vi "CreateLabview.vi"() -> ()   [LabVIEW 2015]
uses:
  Control_Function.ctl
panel:
  in  "Type_Frame":enum16{"SingelCaseFrame", "DoubleCaseFrame"}(ring)=enum."DoubleCaseFrame"
  in  "base path":path=path "D:/control"
  out "String":string
  out "output cluster":T1
  in  "Type_Enum":T2(ring)=enum."Constant"
  in  "Type_Buttom":enum16{"Cluster", "Control", "CheckBox"}(ring)=enum."Control"
  in  "初始化":bool
  in  "Path":path
  in  "初始化歸零?":bool
  in  "Value":string[][](array[string])
  in  "Name":string[](array[string])
  in  "Name_data":string
  in  "Data":string
  in  "檔案格式確認":bool
  in  "路徑修改":bool
  in  "讀出Data":bool
  in  "寫入Data":bool
  in  "結束":bool
  in  "製作框架":bool
  in  "製作按鈕":bool
  in  "儲存CSV":bool
  in  "讀取CSV":bool
  in  "儲存Control":bool
  in  "讀取Control":bool
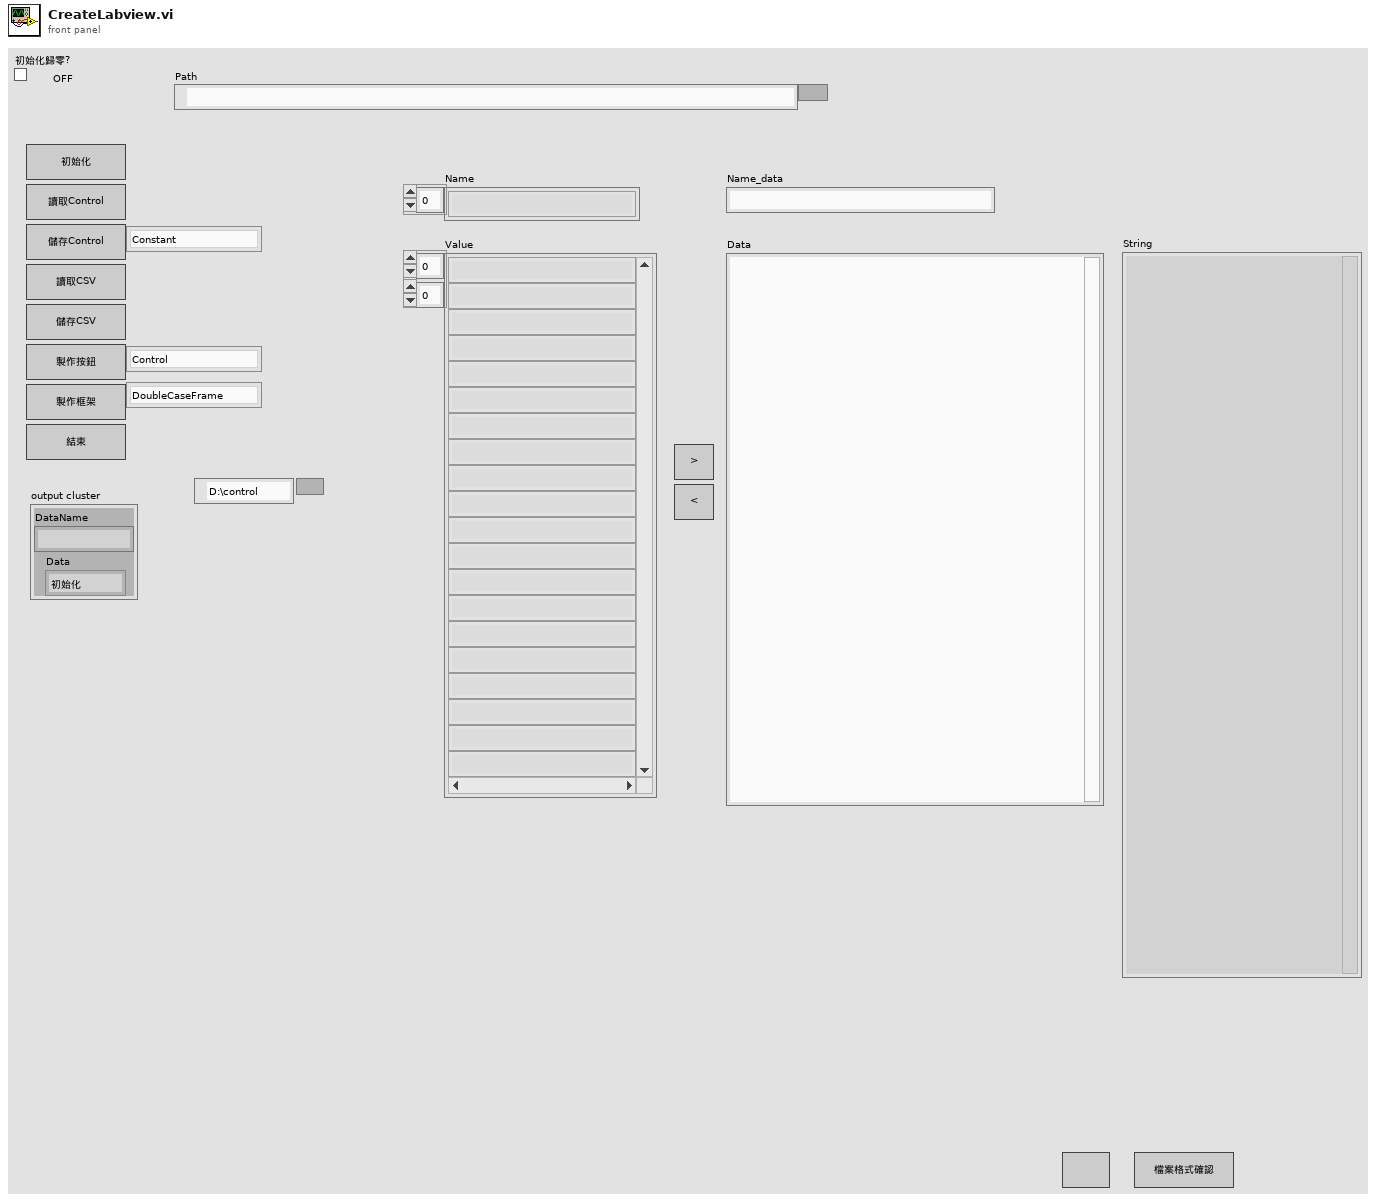
[diagram p1: front panel]
types:
  T1 = cluster{"DataName":string, "Data":enum16{"初始化", "讀取Control", "儲存Control", "讀取CSV", "儲存CSV", "製作按鈕", "製作框架", "結束", "寫入Data", "讀出Data", "路徑修改", "檔案格式確認"}}
  T2 = enum16{"Control", "Constant", "Constant(QMH)", "ClustConstant(QMH)"}
  T3 = typedef "Control_Function.ctl" = cluster{"DataName":string, "Data":enum16{"初始化", "讀取Control", "儲存Control", "讀取CSV", "儲存CSV", "製作按鈕", "製作框架", "資料更新", "寫入Data", "讀出Data", "閒置", "結束"}}
  T4 = enum16{"初始化", "讀取Control", "儲存Control", "讀取CSV", "儲存CSV", "製作按鈕", "製作框架", "結束", "寫入Data", "讀出Data", "路徑修改", "檔案格式確認"}
  T5 = enum16{"初始化", "讀取Control", "儲存Control", "讀取CSV", "儲存CSV", "製作按鈕", "製作框架", "資料更新", "寫入Data", "讀出Data", "閒置", "結束"}
  T6 = cluster{"Alignment":enum32{"Left", "Right", "Hybrid", "Center", "Gravity"}, "Rules":enum32{"Strict", "Allow Wires Under Labels", "Allow Wires Under Lead Nodes", "Allow Wires Under Wide Blocks"}, "Max Heuristic Iterations":u32, "Max Simplex Iterations":u32, "Block Padding":cluster{"Horizontal":i32, "Vertical":i32}, "Wire Padding":cluster{"Horizontal":i32, "Vertical":i32}, "Auto-Tune by Topology":bool, "Fine-Tune Y Positions":bool, "Align All Controls on Left":bool, "Align All Indicators on Right":bool, "Use Array Dimension Heuristics":bool}
  T7 = enum16{"open", "replace", "create", "open or create", "replace or create", "replace or create with confirmation"}
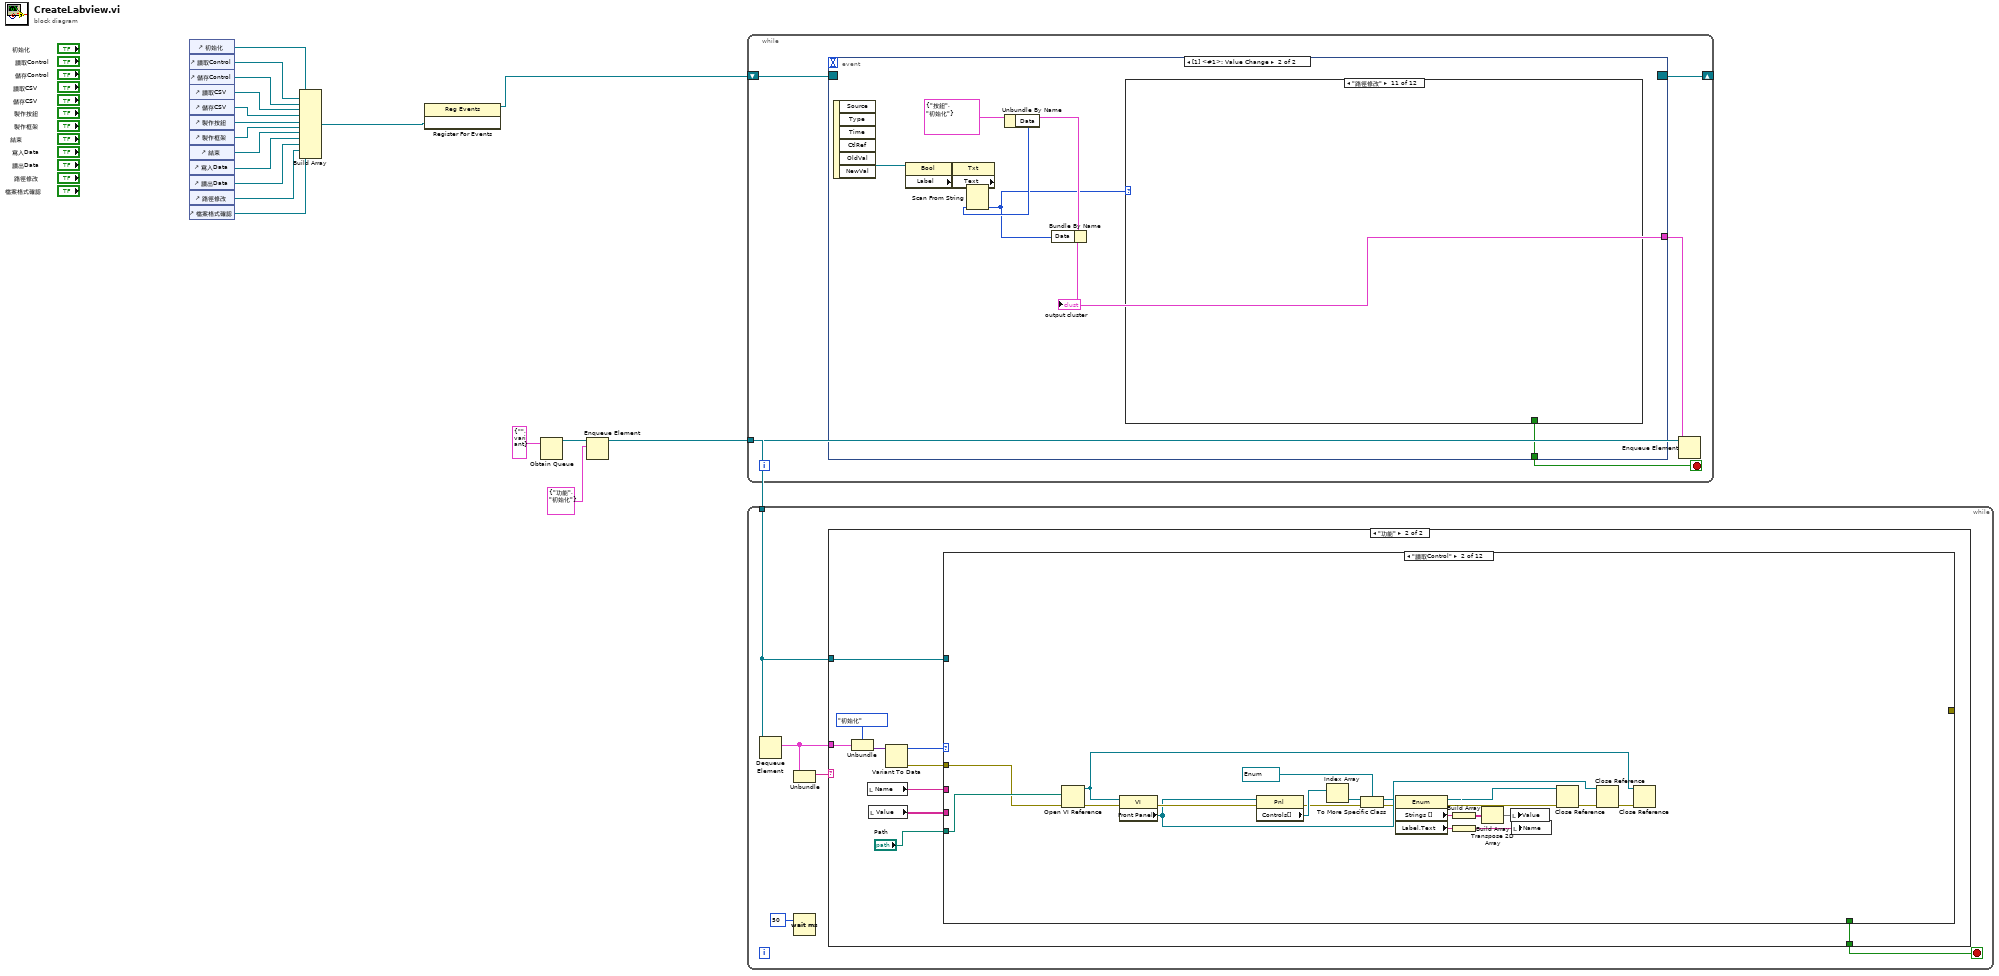
[diagram p0: block diagram]
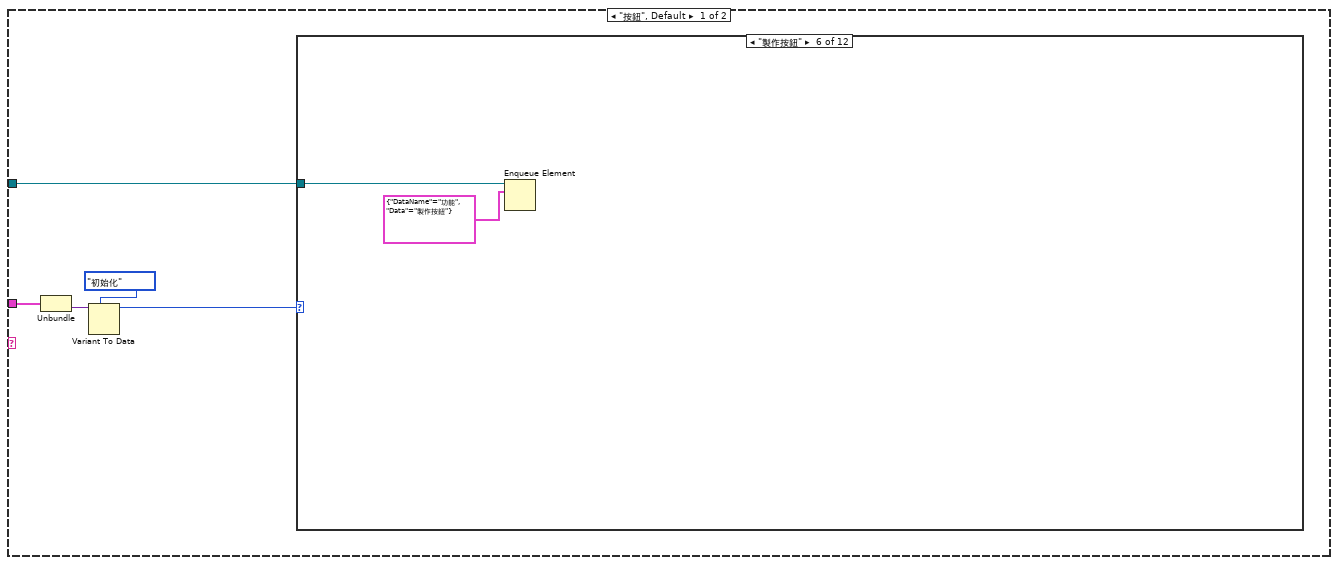
[diagram p2: hidden frame]
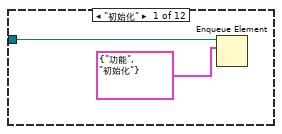
[diagram p3: hidden frame]
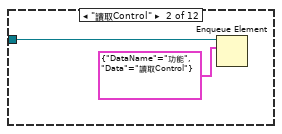
[diagram p4: hidden frame]
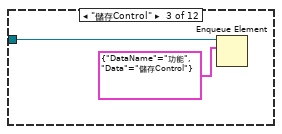
[diagram p5: hidden frame]
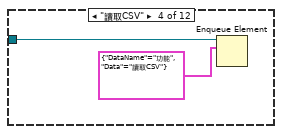
[diagram p6: hidden frame]
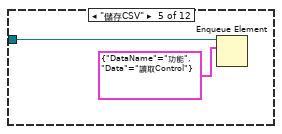
[diagram p7: hidden frame]
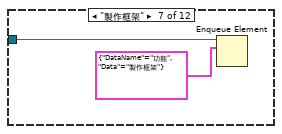
[diagram p8: hidden frame]
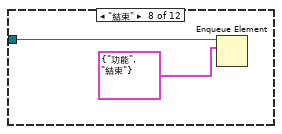
[diagram p9: hidden frame]
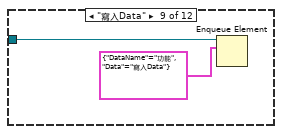
[diagram p10: hidden frame]
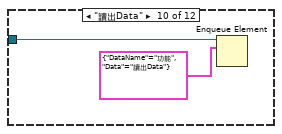
[diagram p11: hidden frame]
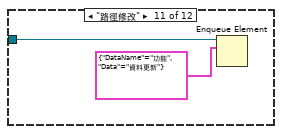
[diagram p12: hidden frame]
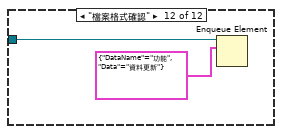
[diagram p13: hidden frame]
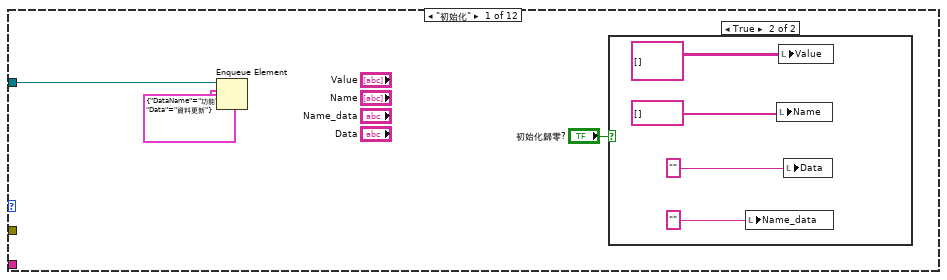
[diagram p14: hidden frame]
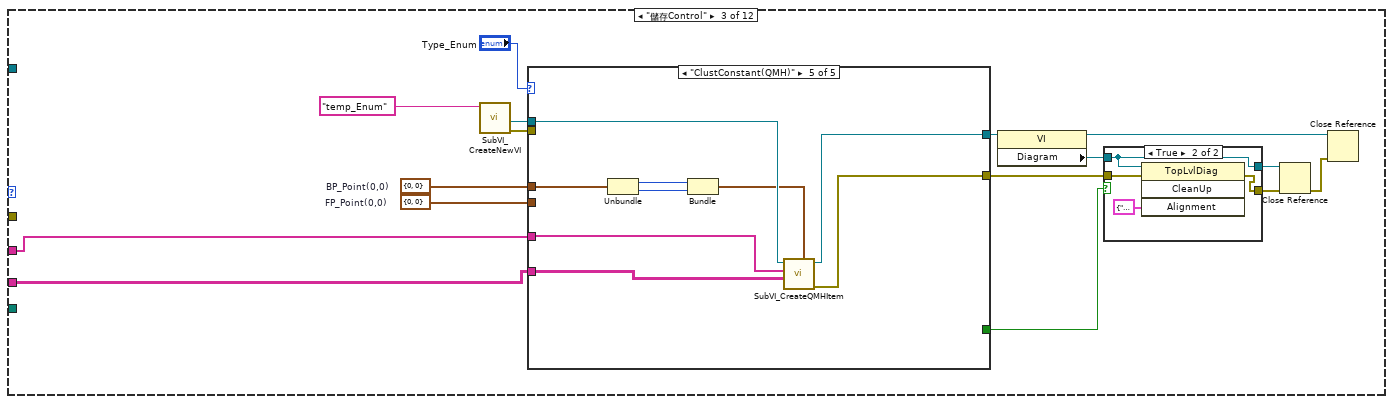
[diagram p16: hidden frame]
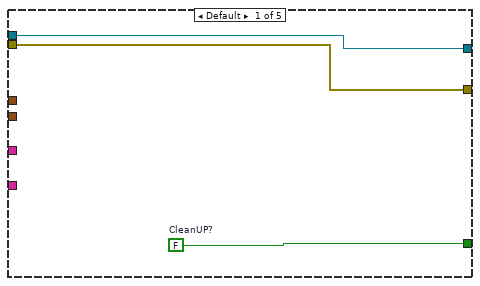
[diagram p18: hidden frame]
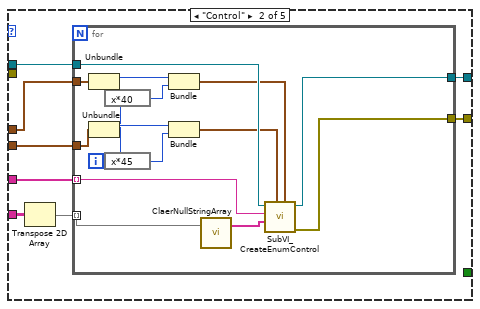
[diagram p19: hidden frame]
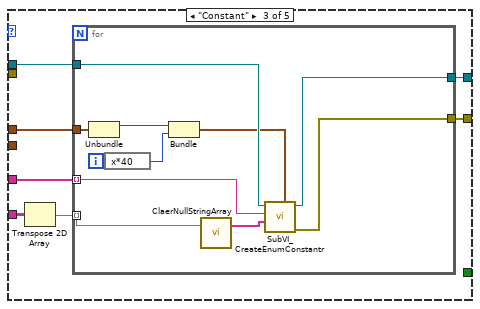
[diagram p20: hidden frame]
diagram:
  n1 = control-ref of="初始化"() -> (w3:refnum<vi>)
  n2 = control-ref of="讀取Control"() -> (w15:refnum<vi>)
  n3 = control-ref of="儲存Control"() -> (w14:refnum<vi>)
  n4 = control-ref of="讀取CSV"() -> (w13:refnum<vi>)
  n5 = control-ref of="儲存CSV"() -> (w12:refnum<vi>)
  n6 = control-ref of="製作按鈕"() -> (w11:refnum<vi>)
  n7 = control-ref of="製作框架"() -> (w10:refnum<vi>)
  n8 = control-ref of="結束"() -> (w1:refnum<vi>)
  n9 = control-ref of="寫入Data"() -> (w9:refnum<vi>)
  n10 = control-ref of="讀出Data"() -> (w8:refnum<vi>)
  n11 = control-ref of="路徑修改"() -> (w7:refnum<vi>)
  n12 = control-ref of="檔案格式確認"() -> (w6:refnum<vi>)
  n13 = Build Array(w3, w15, w14, w13, w12, w11, w10, w1, w9, w8, w7, w6) -> (w2:refnum<vi>[])
  n14 = register-events(w2) -> (reference out=w5:refnum<event-registration>)  [unwired: 2 in, 1 out]
  n15 = Obtain Queue(element data type=cluster{"DataName":string, "DataName":variant} {"DataName"="", "DataName"=variant} ("Cluster")) -> (queue out=w17:refnum<queue>)  [unwired: 4 in, 2 out]
  n16 = Enqueue Element(queue=w17, element=T3 {"DataName"="功能", "Data"=enum."初始化"} ("功能")) -> (queue out=w16:refnum<queue>)  [unwired: 2 in, 2 out]
  n17 = while {
    tunnel: w16 -> [w23]
    shift-right: [w22] -> _
    shift-left: w5 -> [w21]
    stop <- w19 stop-if-true
    n18 = event shown="[1] <#1>: Value Change" {
      selector: w21 -> [_ _]
      dyn-events: [_ _] -> w22
      timeout: _ -> [_ _]
      tunnel: [_ w28] -> w20
      tunnel: [_ w27] -> w19
      event Timeout {
        n19 = event-data() -> ()  [unwired: 1 in, 3 out]
      }
      event Value Change {
        w29 = T1 {"DataName"="按鈕", "Data"=enum."初始化"} ("按鈕")
        n20 = event-data() -> ("CtlRef"=w31:refnum<vi>)  [unwired: 1 in, 5 out]
        n21 = property class="Bool"(reference=w31) -> ("Label"=w30:refnum<vi>)  [unwired: 1 in, 2 out]
        n22 = property class="Txt"(reference=w30) -> ("Text"=w26:string)  [unwired: 1 in, 2 out]
        n23 = Unbundle By Name(w29) -> ("Data"=w25:T4)
        n24 = Scan From String(input string=w26, default 1=w25) -> (output 1=w24:T4)  [unwired: 3 in, 3 out]
        n25 = Bundle By Name(cluster=w29, "Data"=w24) -> (w28:T1)
        "output cluster" <- w28
        n26 = case shown="\"路徑修改\"" w24 {
          tunnel: [_ _ _ _ _ _ _ TRUE _ _ _ _] -> w27
          frame "初始化" {
          }
          frame "讀取Control", Default {
          }
          frame "儲存Control" {
          }
          frame "讀取CSV" {
          }
          frame "儲存CSV" {
          }
          frame "製作按鈕" {
          }
          frame "製作框架" {
          }
          frame "結束" {
          }
          frame "寫入Data" {
          }
          frame "讀出Data" {
          }
          frame "路徑修改" {
          }
          frame "檔案格式確認" {
          }
        }
      }
    }
    n27 = Enqueue Element(queue=w23, element=w20) -> ()  [unwired: 2 in, 3 out]
  }
  n28 = while {
    tunnel: w16 -> [w34]
    stop <- w33 stop-if-true
    n29 = Dequeue Element(queue=w34) -> (element=w35:cluster{"DataName":string, "DataName":variant})  [unwired: 2 in, 3 out]
    n30 = Unbundle(w35) -> ("DataName"=w36:string)  [unwired: 1 out]
    n31 = Wait (ms)(milliseconds to wait=50) -> ()  [unwired: 1 out]
    n32 = case shown="\"功能\"" w36 {
      tunnel: w35 -> [w42 w76]
      tunnel: w34 -> [w39 w72]
      tunnel: [_ w67] -> w33
      frame "按鈕", Default {
        n33 = Unbundle(w42) -> ("DataName"=w41:variant)  [unwired: 1 out]
        n34 = Variant To Data(type=T4."初始化" ("Data"), Variant=w41) -> (data=w40:T4)  [unwired: 1 in, 1 out]
        n35 = case shown="\"製作按鈕\"" w40 {
          tunnel: w39 -> [w43 w46 w47 w49 w51 w53 w55 w57 w59 w61 w63 w65]
          frame "初始化" {
            n36 = Enqueue Element(queue=w43, element=T3 {"DataName"="功能", "Data"=enum."初始化"} ("功能")) -> ()  [unwired: 2 in, 3 out]
          }
          frame "讀取Control" {
            n37 = Enqueue Element(queue=w46, element=T3 {"DataName"="功能", "Data"=enum."讀取Control"} ("功能")) -> ()  [unwired: 2 in, 3 out]
          }
          frame "儲存Control" {
            n38 = Enqueue Element(queue=w47, element=T3 {"DataName"="功能", "Data"=enum."儲存Control"} ("功能")) -> ()  [unwired: 2 in, 3 out]
          }
          frame "讀取CSV" {
            n39 = Enqueue Element(queue=w49, element=T3 {"DataName"="功能", "Data"=enum."讀取CSV"} ("功能")) -> ()  [unwired: 2 in, 3 out]
          }
          frame "儲存CSV" {
            n40 = Enqueue Element(queue=w51, element=T3 {"DataName"="功能", "Data"=enum."讀取Control"} ("功能")) -> ()  [unwired: 2 in, 3 out]
          }
          frame "製作按鈕" {
            n41 = Enqueue Element(queue=w53, element=T3 {"DataName"="功能", "Data"=enum."製作按鈕"} ("功能")) -> ()  [unwired: 2 in, 3 out]
          }
          frame "製作框架" {
            n42 = Enqueue Element(queue=w55, element=T3 {"DataName"="功能", "Data"=enum."製作框架"} ("功能")) -> ()  [unwired: 2 in, 3 out]
          }
          frame "結束" {
            n43 = Enqueue Element(queue=w57, element=T3 {"DataName"="功能", "Data"=enum."結束"} ("功能")) -> ()  [unwired: 2 in, 3 out]
          }
          frame "寫入Data" {
            n44 = Enqueue Element(queue=w59, element=T3 {"DataName"="功能", "Data"=enum."寫入Data"} ("功能")) -> ()  [unwired: 2 in, 3 out]
          }
          frame "讀出Data" {
            n45 = Enqueue Element(queue=w61, element=T3 {"DataName"="功能", "Data"=enum."讀出Data"} ("功能")) -> ()  [unwired: 2 in, 3 out]
          }
          frame "路徑修改" {
            n46 = Enqueue Element(queue=w63, element=T3 {"DataName"="功能", "Data"=enum."資料更新"} ("功能")) -> ()  [unwired: 2 in, 3 out]
          }
          frame "檔案格式確認" {
            n47 = Enqueue Element(queue=w65, element=T3 {"DataName"="功能", "Data"=enum."資料更新"} ("功能")) -> ()  [unwired: 2 in, 3 out]
          }
        }
      }
      frame "功能" {
        n48 = Unbundle(w76) -> ("DataName"=w75:variant)  [unwired: 1 out]
        n49 = local read "Name"() -> (w69:string[])
        n50 = local read "Value"() -> (w68:string[][])
        n51 = Variant To Data(type=T5."初始化" ("功能"), Variant=w75) -> (data=w73:T5, error out=w70:errorcluster)  [unwired: 1 in]
        n52 = case shown="\"讀取Control\"" w73 {
          tunnel: w72 -> [w77 _ _ w199 _ _ _ _ _ _ _ _]
          tunnel: "Path" -> [_ w85 _ w200 w217 _ _ _ _ _ _ _]
          tunnel: w70 -> [_ w84 _ _ w218 w269 _ _ _ _ _ _]
          tunnel: w69 -> [_ _ w106 _ w216 w268 w376 w381 w385 _ _ _]
          tunnel: w68 -> [_ _ w105 _ w215 w267 w375 w380 w386 _ _ _]
          tunnel: [_ _ _ _ w214 w266 _ _ _ _ _ _] -> _
          tunnel: [_ _ _ _ _ _ _ _ _ _ _ TRUE] -> w67
          frame "初始化" {
            n53 = Enqueue Element(queue=w77, element=T3 {"DataName"="功能", "Data"=enum."資料更新"} ("功能")) -> ()  [unwired: 2 in, 3 out]
            n54 = case shown="True" "初始化歸零?" {
              frame False {
              }
              frame True {
                n55 = local write "Name_data"("" ("Data")) -> ()
                n56 = local write "Name"(string[] []) -> ()
                n57 = local write "Value"(string[][] []) -> ()
                n58 = local write "Data"("" ("Data")) -> ()
              }
            }
          }
          frame "讀取Control" {
            n59 = Open VI Reference(vi path=w85, error in (no error)=w84) -> (vi reference=w86:refnum<vi>, error out=w100:errorcluster)  [unwired: 4 in]
            n60 = property class="VI"(reference=w86, error in=w100) -> (error out=w102:errorcluster, "Front Panel"=w101:refnum<vi>)  [unwired: 1 out]
            n61 = property class="Pnl"(reference=w101, error in=w102) -> (error out=w93:errorcluster, "Controls[]"=w99:refnum<vi>[])  [unwired: 1 out]
            n62 = Index Array(array=w99) -> (element=w92:refnum<vi>)  [unwired: 1 in]
            n63 = To More Specific Class(target class=refnum<vi> refnum, reference=w92, error in=w93) -> (specific class reference=w97:refnum<vi>, error out=w95:errorcluster)
            n64 = property class="Enum"(reference=w97, error in=w95) -> (reference out=w96:refnum<vi>, error out=w94:errorcluster, "Strings []"=w91:string[], "Label.Text"=w90:string)
            n65 = Build Array(w91) -> (w88:string[][])
            n66 = Build Array(w90) -> (w89:string[])
            n67 = Transpose 2D Array(2D array=w88) -> (transposed array=w87:string[][])
            n68 = local write "Value"(w87) -> ()
            n69 = local write "Name"(w89) -> ()
            n70 = Close Reference(reference=w96, error in (no error)=w94) -> (error out=w104:errorcluster)
            n71 = Close Reference(reference=w101, error in (no error)=w104) -> (error out=w103:errorcluster)
            n72 = Close Reference(reference=w86, error in (no error)=w103) -> ()  [unwired: 1 out]
          }
          frame "儲存Control" {
            w110 = cluster{"Width":i32, "Height":i32} {"Width"=0, "Height"=0}  # FP_Point(0,0)
            w111 = cluster{"Width":i32, "Height":i32} {"Width"=0, "Height"=0}  # BP_Point(0,0)
            n73 = call "SubVI_CreateNewVI.vi"("vi path"="temp_Enum") -> ("error out"=w108:errorcluster, "VI out"=w109:refnum<vi>)  [unwired: 9 in]
            n74 = case shown="\"ClustConstant(QMH)\"" "Type_Enum" {
              tunnel: w105 -> [_ w134 w159 w174 w196]
              tunnel: w109 -> [w128 w135 w157 w176 w195]
              tunnel: w106 -> [_ w136 w156 w175 w197]
              tunnel: [w128 w133 w155 w173 w194] -> w116
              tunnel: [w127 w132 w154 w172 w193] -> w113
              tunnel: [w129 _ _ _ _] -> w112
              tunnel: w108 -> [w127 _ _ _ _]
              tunnel: w111 -> [_ w130 w153 w171 w191]
              tunnel: w110 -> [_ w131 _ _ _]
              frame Default {
                w129 = FALSE  # CleanUP?
              }
              frame "Control" {
                n75 = Transpose 2D Array(2D array=w134) -> (transposed array=w137:string[][])
                n76 = for {
                  tunnel: w137 -> [w152] mode=indexing
                  tunnel: w135 -> [w151]
                  tunnel: w136 -> [w148] mode=indexing
                  tunnel: [w149] -> w133
                  tunnel: [w147] -> w132
                  tunnel: w131 -> [w144]
                  tunnel: w130 -> [w141]
                  i -> [w140]
                  n77 = Unbundle(w141) -> ("Width"=w143:i32)  [unwired: 1 out]
                  n78 = Unbundle(w144) -> ("Width"=w145:i32)  [unwired: 1 out]
                  n79 = expression code="x*40"(w140) -> (w142:i32)
                  n80 = expression code="x*45"(w140) -> (w146:i32)
                  n81 = Bundle("Width"=w143, w142) -> (w139:cluster{"Width":i32, i32})  [unwired: 1 in]
                  n82 = Bundle("Width"=w145, w146) -> (w138:cluster{"Width":i32, i32})  [unwired: 1 in]
                  n83 = call <userlib>:"ClaerNullStringArray.vi"("Array in"=w152) -> ("Array out"=w150:string[])  [unwired: 18 in]
                  n84 = call <userlib>:"SubVI_CreateEnumControl.vi"("BP_Point(0,0)"=w139, "FP_Point(0,0)"=w138, "Value"=w150, "Name"=w148, "VI in"=w151) -> ("error out"=w147:errorcluster, "VI out"=w149:refnum<vi>)  [unwired: 4 in, 1 out]
                }
              }
              frame "Constant" {
                n85 = Transpose 2D Array(2D array=w159) -> (transposed array=w158:string[][])
                n86 = for {
                  tunnel: w158 -> [w170] mode=indexing
                  tunnel: w157 -> [w169]
                  tunnel: w156 -> [w166] mode=indexing
                  tunnel: [w168] -> w155
                  tunnel: [w165] -> w154
                  tunnel: w153 -> [w164]
                  i -> [w163]
                  n87 = Unbundle(w164) -> ("Width"=w160:i32)  [unwired: 1 out]
                  n88 = expression code="x*40"(w163) -> (w161:i32)
                  n89 = Bundle("Width"=w160, w161) -> (w162:cluster{"Width":i32, i32})  [unwired: 1 in]
                  n90 = call <userlib>:"ClaerNullStringArray.vi"("Array in"=w170) -> ("Array out"=w167:string[])  [unwired: 18 in]
                  n91 = call "SubVI_CreateEnumConstantr.vi"("BP_Point(0,0)"=w162, "Value"=w167, "Name"=w166, "VI in"=w169) -> ("error out"=w165:errorcluster, "VI out"=w168:refnum<vi>)  [unwired: 6 in]
                }
              }
              frame "Constant(QMH)" {
                n92 = Transpose 2D Array(2D array=w174) -> (transposed array=w177:string[][])
                n93 = for {
                  tunnel: w177 -> [w188] mode=indexing
                  tunnel: w176 -> [w187]
                  tunnel: w175 -> [w186] mode=indexing
                  tunnel: [w184] -> w173
                  tunnel: [w183] -> w172
                  tunnel: w171 -> [w182]
                  i -> [w181]
                  n94 = Unbundle(w182) -> ("Width"=w178:i32)  [unwired: 1 out]
                  n95 = call <userlib>:"ClaerNullStringArray.vi"("Array in"=w188) -> ("Array out"=w185:string[])  [unwired: 18 in]
                  n96 = expression code="x*16"(w181) -> (w179:i32)
                  n97 = Bundle("Width"=w178, w179) -> (w180:cluster{"Width":i32, i32})  [unwired: 1 in]
                  n98 = call "SubVI_CreateEnumCluster.vi"("BP_Point(0,0)"=w180, "Data"=w185, "Name"=w186, "VI in"=w187) -> ("error out"=w183:errorcluster, "VI out"=w184:refnum<vi>)  [unwired: 5 in, 1 out]
                }
              }
              frame "ClustConstant(QMH)" {
                n99 = Unbundle(w191) -> ("Width"=w190:i32, "Height"=w192:i32)
                n100 = Bundle("Width"=w190, "Height"=w192) -> (w189:cluster{"Width":i32, "Height":i32})  [unwired: 1 in]
                n101 = call "SubVI_CreateQMHItem.vi"("BP_Point(0,0)"=w189, "Value"=w196, "Name"=w197, "VI in"=w195) -> ("error out"=w193:errorcluster, "VI out"=w194:refnum<vi>)  [unwired: 6 in]
              }
            }
            n102 = property on="Property Node" class="VI"(reference=w116) -> (reference out=w114:refnum<vi>, "Diagram"=w115:refnum<vi>)  [unwired: 1 in, 1 out]
            n103 = case shown="True" w112 {
              tunnel: [w122 w123] -> w120
              tunnel: [w121 w126] -> w119
              tunnel: w115 -> [w122 w123]
              tunnel: w113 -> [w121 w124]
              frame False {
              }
              frame True {
                n104 = invoke class="TopLvlDiag" method="CleanUp"(reference=w123, error in=w124, "Alignment"=T6 {"Alignment"=enum."Left", "Rules"=enum."Strict", "Max Heuristic Iterations"=0, "Max Simplex Iterations"=0, "Block Padding"={"Horizontal"=0, "Vertical"=0}, "Wire Padding"={"Horizontal"=0, "Vertical"=0}, "Auto-Tune by Topology"=FALSE, "Fine-Tune Y Positions"=FALSE, "Align All Controls on Left"=FALSE, "Align All Indicators on Right"=FALSE, "Use Array Dimension Heuristics"=FALSE} ("Clean Up Options")) -> (error out=w126:errorcluster)  [unwired: 1 in, 3 out]
              }
            }
            n105 = Close Reference(reference=w120, error in (no error)=w119) -> (error out=w118:errorcluster)
            n106 = Close Reference(reference=w114, error in (no error)=w118) -> ()  [unwired: 1 out]
          }
          frame "讀取CSV" {
            w204 = 0 ("index")
            n107 = Enqueue Element(queue=w199, element=T3 {"DataName"="功能", "Data"=enum."資料更新"} ("功能")) -> ()  [unwired: 2 in, 3 out]
            n108 = Open/Create/Replace File(file path (use dialog)=w200) -> (refnum out=w213:refnum<file>, error out=w207:errorcluster)  [unwired: 5 in, 1 out]
            n109 = Read from Text File(file (use dialog)=w213, error in=w207) -> (refnum out=w209:refnum<file>, text=w211:string, error out=w208:errorcluster)  [unwired: 2 in, 1 out]
            n110 = Close File(refnum=w209, error in=w208) -> ()  [unwired: 2 out]
            n111 = Spreadsheet String To Array(delimiter (Tab)=",", format string="%s" ("delimiter (\\t)"), spreadsheet string=w211, array type (2D Dbl)=string[][] [] ("Array")) -> (array=w206:string[][])
            n112 = Array Subset(array=w206, index (row)=w204, index (col)=w204) -> ()  [unwired: 2 in, 1 out]
            n113 = Delete From Array(array=w206, index (row)=0) -> (deleted portion=w203:string[], array with subset deleted=w202:string[][])  [unwired: 2 in]
            n114 = local write "Name"(w203) -> ()
            n115 = local write "Value"(w202) -> ()
          }
          frame "儲存CSV" {
            n116 = Build Array (concatenate)(w216, w215) -> (w223:string[][])
            n117 = for {
              tunnel: w223 -> [w244] mode=indexing
              shift-right: [w240] -> w225
              shift-left: "" -> [w241]
              tunnel: [w237] -> w224
              tunnel: w218 -> [w235]
              i -> [w239]
              n118 = for {
                tunnel: w244 -> [w258] mode=indexing
                shift-right: [w256] -> w242
                shift-left: "" -> [w257]
                tunnel: [w253] -> w236
                tunnel: w235 -> [w252]
                i -> [w255]
                n119 = Not Equal To 0?(x=w255) -> (x != 0?=w254:bool)
                n120 = case shown="False" w254 {
                  tunnel: w258 -> [w260 w264]
                  tunnel: w257 -> [_ w263]
                  tunnel: [w260 w262] -> w256
                  tunnel: [w259 w261] -> w253
                  tunnel: w252 -> [w259 w261]
                  frame False {
                  }
                  frame True {
                    n121 = Concatenate Strings(w263, ",", w264) -> (w262:string)
                  }
                }
              }
              n122 = Not Equal To 0?(x=w239) -> (x != 0?=w238:bool)
              n123 = case shown="False" w238 {
                tunnel: w242 -> [w246 w251]
                tunnel: w241 -> [_ w249]
                tunnel: [w246 w248] -> w240
                tunnel: [w245 w247] -> w237
                tunnel: w236 -> [w245 w247]
                frame False {
                }
                frame True {
                  n124 = Concatenate Strings(w249, "\r", w251) -> (w248:string)
                }
              }
            }
            n125 = Two Button Dialog(message="是否存檔?") -> (T button?=w221:bool)  [unwired: 2 in]
            n126 = case shown="True" w221 {
              tunnel: T7."open or create" ("operation (0:open)") -> [_ w233]
              tunnel: w225 -> [_ w232]
              tunnel: [w226 w229] -> w214
              tunnel: w217 -> [_ w227]
              tunnel: w224 -> [w226 _]
              frame False {
              }
              frame True {
                n127 = Open/Create/Replace File(file path (use dialog)=w227, operation (0:open)=w233) -> (refnum out=w234:refnum<file>, error out=w228:errorcluster)  [unwired: 4 in, 1 out]
                n128 = Write to Text File(file (use dialog)=w234, text=w232, error in=w228) -> (refnum out=w230:refnum<file>, error out=w231:errorcluster)  [unwired: 1 in, 1 out]
                n129 = Close File(refnum=w230, error in=w231) -> (error out=w229:errorcluster)  [unwired: 1 out]
              }
            }
          }
          frame "製作按鈕" {
            w280 = cluster{"Width":i32, "Height":i32} {"Width"=0, "Height"=0}  # FP_Point(0,0)
            w279 = cluster{"Width":i32, "Height":i32} {"Width"=0, "Height"=0}  # BP_Point(0,0)
            n130 = Transpose 2D Array(2D array=w267) -> (transposed array=w281:string[][])
            n131 = call "SubVI_CreateNewVI.vi"("error in (no error)"=w269, "vi path"="temp_Buttom") -> ("error out"=w283:errorcluster, "VI out"=w285:refnum<vi>)  [unwired: 8 in]
            n132 = for {
              tunnel: w285 -> [w306]
              tunnel: w283 -> [w308]
              tunnel: [w307] -> w272
              tunnel: w281 -> [w304] mode=indexing
              tunnel: w268 -> [w305] mode=indexing
              tunnel: "Type_Buttom" -> [w303]
              tunnel: w280 -> [w302]
              tunnel: w279 -> [w299]
              tunnel: [w301] -> w277
              tunnel: [w300] -> w270
              i -> [w296]
              n133 = expression code="x*300"(w296) -> (w295:i32)
              n134 = Unbundle(w299) -> ("Width"=w294:i32, "Height"=w297:i32)
              n135 = Add(x=w295, y=w294) -> (x+y=w293:i32)
              n136 = Bundle(w293, "Height"=w297) -> (w298:cluster{i32, "Height":i32})  [unwired: 1 in]
              n137 = case shown="\"CheckBox\"" w303 {
                tunnel: w308 -> [w324 w332 w357 w370]
                tunnel: [w327 w332 w349 w369] -> w307
                tunnel: w306 -> [w326 w333 w347 w359]
                tunnel: w305 -> [w329 _ _ w358]
                tunnel: w304 -> [w331 _ w356 w372]
                tunnel: w296 -> [w320 _ w355 w366]
                tunnel: w302 -> [w316 _ w341 w362]
                tunnel: w298 -> [w317 _ w343 w361]
                tunnel: [w325 w333 w346 w360] -> w301
                tunnel: [_ w334 _ _] -> w300
                frame "Cluster" {
                  n138 = call <userlib>:"ClaerNullStringArray.vi"("Array in"=w331) -> ("Array out"=w312:string[])  [unwired: 18 in]
                  n139 = expression code="x*110"(w320) -> (w322:i32)
                  n140 = Bundle(w322, 0) -> (w321:cluster{i32, i32})  [unwired: 1 in]
                  n141 = Array Size(array=w312) -> (size(s)=w314:i32)
                  n142 = expression code="x*6"(w314) -> (w313:i32)
                  n143 = Add(x=w321, y=w317) -> (x+y=w318:cluster{i32, i32})
                  n144 = Add(x=w321, y=w316) -> (x+y=w315:cluster{i32, i32})
                  n145 = call "SubVI_CreateBottomCluster.vi"("BP_Point(0,0)"=w318, "Ref位移"=150, "FP_Point(0,0)"=w315, "error in (no error)"=w324, "Value"=w312, "Name"=w329, "VI in"=w326) -> ("Array"=w328:refnum<vi>[], "VI out"=w330:refnum<vi>)  [unwired: 2 in, 1 out]
                  n146 = Bundle(230, w313) -> (w311:cluster{i32, i32})  [unwired: 1 in]
                  n147 = Add(x=w318, y=w311) -> (x+y=w323:cluster{i32, i32})
                  n148 = call "SubVI_CreateBuildArray.vi"("BP_Point(0,0)"=w323, "Array"=w328, "VI in"=w330) -> ("error out"=w327:errorcluster, "VI out"=w325:refnum<vi>)  [unwired: 6 in, 1 out]
                }
                frame Default {
                  w334 = FALSE  # CleanUP?
                }
                frame "Control" {
                  n149 = call <userlib>:"ClaerNullStringArray.vi"("Array in"=w356) -> ("Array out"=w340:string[])  [unwired: 18 in]
                  n150 = expression code="x*110"(w355) -> (w354:i32)
                  n151 = Bundle(w354, 0) -> (w342:cluster{i32, i32})  [unwired: 1 in]
                  n152 = Array Size(array=w340) -> (size(s)=w339:i32)
                  n153 = expression code="x*6"(w339) -> (w337:i32)
                  n154 = Add(x=w342, y=w343) -> (x+y=w345:cluster{i32, i32})
                  n155 = Add(x=w342, y=w341) -> (x+y=w344:cluster{i32, i32})
                  n156 = call "SubVI_CreateBottom.vi"("BP_Point(0,0)"=w345, "Ref位移"=150, "FP_Point(0,0)"=w344, "error in (no error)"=w357, "Value"=w340, "VI in"=w347) -> ("error out"=w350:errorcluster, "Array"=w352:refnum<vi>[], "VI out"=w353:refnum<vi>)  [unwired: 3 in]
                  n157 = Bundle(230, w337) -> (w336:cluster{i32, i32})  [unwired: 1 in]
                  n158 = Add(x=w345, y=w336) -> (x+y=w351:cluster{i32, i32})
                  n159 = call "SubVI_CreateBuildArray.vi"("BP_Point(0,0)"=w351, "error in (no error)"=w350, "Array"=w352, "VI in"=w353) -> ("error out"=w349:errorcluster, "VI out"=w346:refnum<vi>)  [unwired: 5 in, 1 out]
                }
                frame "CheckBox" {
                  n160 = call <userlib>:"ClaerNullStringArray.vi"("Array in"=w372) -> ("Array out"=w371:string[])  [unwired: 18 in]
                  n161 = expression code="x*600"(w366) -> (w368:i32)
                  n162 = Bundle(w368, 0) -> (w367:cluster{i32, i32})  [unwired: 1 in]
                  n163 = Add(x=w367, y=w361) -> (x+y=w363:cluster{i32, i32})
                  n164 = Add(x=w367, y=w362) -> (x+y=w364:cluster{i32, i32})
                  n165 = call "SubVI_CreateCheckBoxCluster.vi"("BP_Point(0,0)"=w363, "FP_Point(0,0)"=w364, "error in (no error)"=w370, "Value"=w371, "Name"=w358, "VI In"=w359) -> ("error out"=w369:errorcluster, "VI out"=w360:refnum<vi>)  [unwired: 4 in]
                }
              }
            }
            n166 = property on="Property Node" class="VI"(reference=w277, error in=w272) -> (reference out=w278:refnum<vi>, error out=w275:errorcluster, "Diagram"=w276:refnum<vi>)
            n167 = case shown="True" w270 {
              tunnel: w276 -> [w287 w291]
              tunnel: w275 -> [w286 w290]
              tunnel: [w286 w289] -> w274
              tunnel: [w287 w288] -> w271
              frame False {
              }
              frame True {
                n168 = invoke class="TopLvlDiag" method="CleanUp"(reference=w291, error in=w290, "Alignment"=T6 {"Alignment"=enum."Left", "Rules"=enum."Strict", "Max Heuristic Iterations"=0, "Max Simplex Iterations"=0, "Block Padding"={"Horizontal"=0, "Vertical"=0}, "Wire Padding"={"Horizontal"=0, "Vertical"=0}, "Auto-Tune by Topology"=FALSE, "Fine-Tune Y Positions"=FALSE, "Align All Controls on Left"=TRUE, "Align All Indicators on Right"=TRUE, "Use Array Dimension Heuristics"=FALSE} ("Clean Up Options")) -> (reference out=w288:refnum<vi>, error out=w289:errorcluster)  [unwired: 1 in, 2 out]
              }
            }
            n169 = Close Reference(reference=w271, error in (no error)=w274) -> (error out=w273:errorcluster)
            n170 = Close Reference(reference=w278, error in (no error)=w273) -> (error out=w266:errorcluster)
          }
          frame "製作框架" {
            n171 = case shown="\"DoubleCaseFrame\"" "Type_Frame" {
              tunnel: w376 -> [_ w379]
              tunnel: w375 -> [_ w378]
              tunnel: "base path" -> [_ w377]
              frame "SingelCaseFrame", Default {
              }
              frame "DoubleCaseFrame" {
                n172 = call "formge.vi"("base path"=w377, "Message Data"=w378, "Message"=w379) -> ()  [unwired: 9 in]
              }
            }
          }
          frame "資料更新" {
            n173 = call "SubVI_ConvertToDataString.vi"("Data"=w380, "DataName"=w381) -> ("DataString"=→"String":string)  [unwired: 8 in, 1 out]
          }
          frame "寫入Data" {
            n174 = for {
              tunnel: w386 -> [w405] mode=indexing
              shift-right: [w401] -> w383
              shift-left: "" -> [w402]
              i -> [w400]
              n175 = for {
                tunnel: w405 -> [w415] mode=indexing
                shift-right: [w413] -> w403
                shift-left: "" -> [w414]
                i -> [w411]
                n176 = Not Equal To 0?(x=w411) -> (x != 0?=w412:bool)
                n177 = case shown="True" w412 {
                  tunnel: w415 -> [w416 w419]
                  tunnel: w414 -> [_ w417]
                  tunnel: [w416 w418] -> w413
                  frame False {
                  }
                  frame True {
                    n178 = Concatenate Strings(w417, ",", w419) -> (w418:string)
                  }
                }
              }
              n179 = Not Equal To 0?(x=w400) -> (x != 0?=w399:bool)
              n180 = case shown="True" w399 {
                tunnel: w403 -> [w406 w410]
                tunnel: w402 -> [_ w408]
                tunnel: [w406 w407] -> w401
                frame False {
                }
                frame True {
                  n181 = Concatenate Strings(w408, "\r", w410) -> (w407:string)
                }
              }
            }
            n182 = for {
              tunnel: w385 -> [w393] mode=indexing
              shift-right: [w391] -> w384
              shift-left: "" -> [w392]
              i -> [w389]
              n183 = Not Equal To 0?(x=w389) -> (x != 0?=w390:bool)
              n184 = case shown="True" w390 {
                tunnel: w393 -> [w394 w397]
                tunnel: w392 -> [_ w395]
                tunnel: [w394 w396] -> w391
                frame False {
                }
                frame True {
                  n185 = Concatenate Strings(w395, ",", w397) -> (w396:string)
                }
              }
            }
            n186 = local write "Name_data"(w384) -> ()
            n187 = local write "Data"(w383) -> ()
          }
          frame "讀出Data" {
            (unwired) "\r"
            n188 = local read "Name_data"() -> (w424:string)
            n189 = local read "Data"() -> (w425:string)
            n190 = Spreadsheet String To Array(format string="%s", spreadsheet string=w425, array type (2D Dbl)=string[][] []) -> (array=w432:string[][])  [unwired: 1 in]
            n191 = Index Array(array=w432, index (col)=0 ("disabled index (col)")) -> (element=w430:string[])  [unwired: 1 in]
            n192 = for {
              tunnel: w430 -> [w437] mode=indexing
              tunnel: [w435] -> w423 mode=indexing
              n193 = Spreadsheet String To Array(delimiter (Tab)="," ("format string"), format string="%s", spreadsheet string=w437, array type (2D Dbl)=string[][] []) -> (array=w434:string[][])
              n194 = Index Array(array=w434) -> (element=w435:string[])  [unwired: 2 in]
            }
            n195 = Spreadsheet String To Array(delimiter (Tab)="," ("format string"), format string="%s", spreadsheet string=w424, array type (2D Dbl)=string[][] []) -> (array=w429:string[][])
            n196 = Index Array(array=w429) -> (element=w422:string[])  [unwired: 2 in]
            n197 = local write "Value"(w423) -> ()
            n198 = local write "Name"(w422) -> ()
          }
          frame "閒置" {
          }
          frame "結束" {
          }
        }
      }
    }
  }
